vi "Connection Callback.vi"(7 "Owner":refnum<class>, 8 "error in (no error)":errorcluster, 10 "Connection State":T1, 11 "Connection":refnum<class "Connection.lvclass">) -> (0 "error out":errorcluster)   [LabVIEW 2020, in "HTTP Server.lvlib" / "Server.lvclass"]
uses:
  Server.lvclass
  <vilib>/IlluminatedG/lv-stream/Connection/Connection.lvclass
  <vilib>/IlluminatedG/lv-stream/Connection State.ctl
  Server.lvclass/Server.ctl
  <vilib>/IlluminatedG/lv-stream/Stream.lvlib
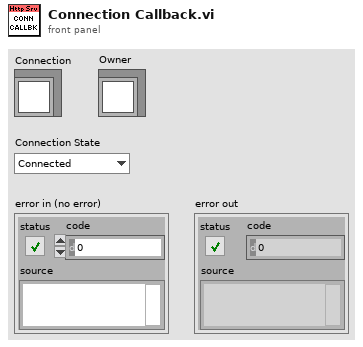
[diagram p1: front panel]
types:
  T1 = typedef "Stream.lvlib/Connection State.ctl" = enum16{"Connected", "Disconnected"}
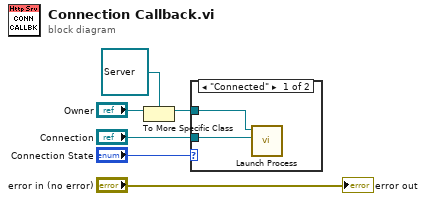
[diagram p0: block diagram]
diagram:
  n1 = To More Specific Class(target class=refnum<class "Server.lvclass"> refnum ("HTTP.lvlib:Server.lvclass"), reference="Owner") -> (specific class reference=w3:refnum<class "Server.lvclass">)  [unwired: 1 in, 1 out]
  n2 = case shown="\"Connected\"" "Connection State" {
    tunnel: w3 -> [w8 _]
    tunnel: "Connection" -> [w7 _]
    frame "Connected" {
      n3 = call "Launch Process.vi"("Connection"=w7, "Server in"=w8) -> ()  [unwired: 8 in, 2 out]
    }
    frame "Disconnected" {
    }
  }
  "error out" <- "error in (no error)"
